vi "Write Key Value Boolean.vi"(7 "Section Name":string, 8 "error in (no error)":errorcluster, 9 "Value":bool, 10 "Key Name":string, 11 "ODBC-Interface in":refnum<class "ODBC-Interface.lvclass">) -> (0 "error out":errorcluster, 2 "found":bool, 3 "ODBC-Interface out":refnum<class "ODBC-Interface.lvclass">)   [LabVIEW 2016, in "DB-Configuration.lvlib" / "ODBC-Interface.lvclass"]
doc: "Write boolean key value."
uses:
  ODBC-Interface.lvclass
  Configuration/Classes/Section/Section.lvclass
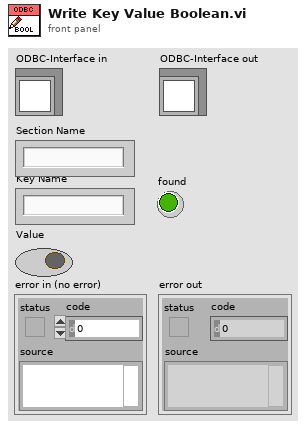
[diagram p1: front panel]
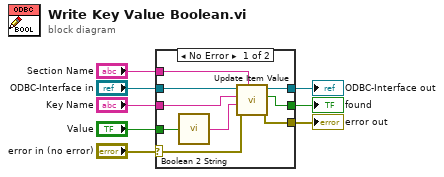
[diagram p0: block diagram]
diagram:
  n1 = case shown="No Error" "error in (no error)" {
    selector: "error in (no error)" -> [w9 w18]
    tunnel: "Section Name" -> [w17 _]
    tunnel: "ODBC-Interface in" -> [w16 w19]
    tunnel: [w15 w19] -> w6
    tunnel: "Key Name" -> [w14 _]
    tunnel: "Value" -> [w13 _]
    tunnel: [w11 w18] -> w3
    tunnel: [w10 _] -> w2
    frame No Error {
      n2 = call "Boolean 2 String.vi"("Boolean"=w13) -> ("Boolean String"=w12:string)
      n3 = call-dynamic "Update Item Value.vi"("Section Name"=w17, "error in (no error)"=w9, "Value"=w12, "Key Name"=w14, "ODBC-Interface in"=w16) -> ("error out"=w11:errorcluster, "found"=w10:bool, "ODBC-Interface out"=w15:refnum<class "ODBC-Interface.lvclass">)  [unwired: 4 in]
    }
    frame Error {
    }
  }
  "error out" <- w3
  "ODBC-Interface out" <- w6
  "found" <- w2
